vi "S2C_ErrorTrap.vi"(8 "Error In":errorcluster) -> (0 "Error Out":errorcluster)   [LabVIEW 2015]
doc: "Detects an error and calls the error case to process the error."
uses:
  Globals/S2C_Globals.vi
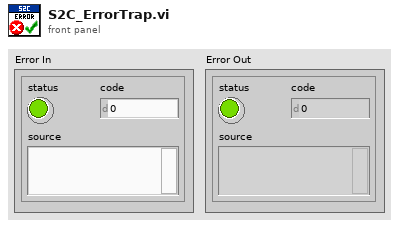
[diagram p1: front panel]
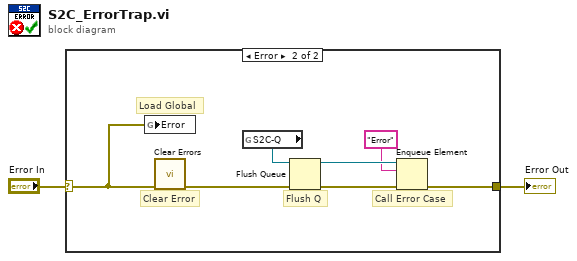
[diagram p0: block diagram]
diagram:
  n1 = case shown="Error" "Error In" {
    selector: "Error In" -> [w3 w10]
    tunnel: [w3 w4] -> w1
    frame No Error {
    }
    frame Error {
      # "Load Global"
      # "Call Error Case"
      # "Flush Q"
      # "Clear Error"
      n2 = global write "S2C_Globals.vi" "Error"(w10) -> ()
      n3 = call <vilib>:"Clear Errors.vi"("error in (no error)"=w10) -> ("error out"=w9:errorcluster)  [unwired: 5 in, 1 out]
      n4 = global read "S2C_Globals.vi" "S2C-Q"() -> (w8:refnum<queue>)
      n5 = Flush Queue(queue=w8, error in (no error)=w9) -> (queue out=w6:refnum<queue>, error out=w7:errorcluster)  [unwired: 1 out]
      n6 = Enqueue Element(queue=w6, element="Error", error in (no error)=w7) -> (error out=w4:errorcluster)  [unwired: 1 in, 2 out]
    }
  }
  "Error Out" <- w1
